vi "Initialise bleaching compensation.vi"(8 "error in (no error)":errorcluster, 11 "RSA in":refnum<class "RSA.lvclass">) -> (0 "error out":errorcluster, 3 "RSA out":refnum<class "RSA.lvclass">)   [LabVIEW 2012, in "RSA.lvclass"]
uses:
  RSA.lvclass
  <vilib>/Distrio/Murmex/GenericMessage/GenericMessage.lvclass
  <vilib>/Distrio/Murmex/Message/Add or replace parameter.vi
  <vilib>/Distrio/Murmex/Murmex/Murmex.lvclass
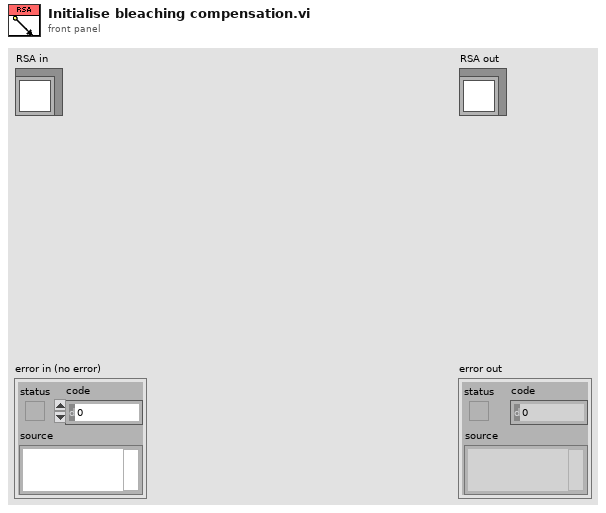
[diagram p1: front panel]
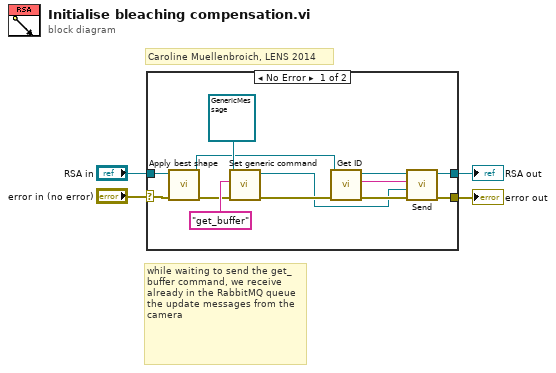
[diagram p0: block diagram]
diagram:
  # "while waiting to send the get_buffer command, we receive already in the RabbitMQ queue the update messages from the camera"
  # "Caroline Muellenbroich, LENS 2014"
  n1 = case shown="No Error" "error in (no error)" {
    selector: "error in (no error)" -> [w15 w19]
    tunnel: [w12 w19] -> w3
    tunnel: [w11 w18] -> w1
    tunnel: "RSA in" -> [w13 w18]
    frame No Error {
      n2 = call "Apply best shape.vi"("error in (no error)"=w15, "RSA in"=w13) -> ("error out"=w14:errorcluster, "RSA out"=w10:refnum<class "RSA.lvclass">)  [unwired: 8 in]
      n3 = call <vilib>:"Set generic command.vi"("error in (no error)"=w14, "generic command"="get_buffer", "GenericMessage in"=refnum<class "GenericMessage.lvclass"> refnum ("Murmex.lvlib:GenericMessage")) -> ("error out"=w8:errorcluster, "GenericMessage out"=w5:refnum<class "GenericMessage.lvclass">)  [unwired: 7 in]
      n4 = call <vilib>:"Get ID.vi"("error in (no error)"=w8, "Murmex in"=w10) -> ("error out"=w7:errorcluster, "component id"=w6:string, "Murmex out"=w9:refnum<class "RSA.lvclass">)  [unwired: 7 in]
      n5 = call <vilib>:"Send.vi"("error in (no error)"=w7, "Message"=w5, "recipient"=w6, "Murmex in"=w9) -> ("error out"=w12:errorcluster, "Murmex out"=w11:refnum<class "RSA.lvclass">)  [unwired: 6 in]
    }
    frame Error {
    }
  }
  "error out" <- w3
  "RSA out" <- w1
